vi "FRIC_navX_Internal_Serial_ProcessingLoop.vi"(7 "Device Number":T1, 9 "Stream Type":T2=enum."AHRSAndPositioning", 10 "Serial Port":T3=enum."MXP TTL", 11 "Update Rate (4Hz-200Hz)":u8=50 min=4 max=200) -> ()   [LabVIEW 2015]
doc: "This navX VI handles the reading/writing for the navX. All of the good stuff is in here.\nTHIS VI SHOULD NOT BE CALLED BY THE USER!"
uses:
  _NI WPI Serial USB/WPI_SerialPort_USB.ctl
  _TypeDefs/Z900_navX_SerialStreamTypeDef.ctl
  _TypeDefs/FRIC_navX_DeviceNumbersTypeDef.ctl
  _TypeDefs/FRIC_navX_I2C Process Loop TypeDef.ctl
  _TypeDefs/FRIC_navX_ProcessingLoopStatesTypeDef_I2C.ctl
  _TypeDefs/Z900_navX_DeviceTypeDef.ctl
  _TypeDefs/Z900_navX_ProtocolTypeDef.ctl
  _TypeDefs/Z900_navX_NotifyPacketTypeDef.ctl
  _TypeDefs/Z900_navX_ActionTypeDef.ctl
  <vilib>/Rock Robotics/SystemInterfaces/i2clib/i2c_bus.ctl
  _TypeDefs/Z900_navX_IntegrationControlRegisters.ctl
  <vilib>/Rock Robotics/WPI/SPI/WPI_SPIDevRef.ctl
  <vilib>/Rock Robotics/SystemInterfaces/spilib/spi_bus.ctl
  <vilib>/Rock Robotics/WPI/SerialPort/WPI_SerialPortRef.ctl
  _Device/_Internal/SERIAL/Z900_navX_SERIAL_ValidatePacketChecksum.vi
  _Device/_Internal/SERIAL/Z900_navX_SERIAL_ValidatePacketTermination.vi
  <vilib>/Rock Robotics/SystemInterfaces/Utilities/FPGA_UtilitiesRead LocalTime.vi
  _NI WPI Serial USB/_NI WPI Serial USB.lvlib
panel:
  out "Loop Time (ms)":dbl
  out "Connected":bool
  in  "Halt":bool
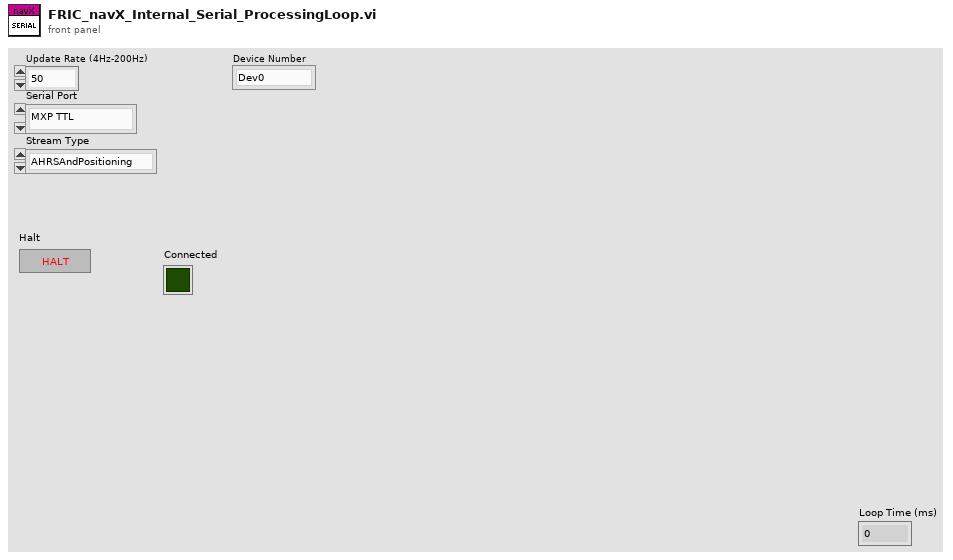
[diagram p1: front panel]
types:
  T1 = typedef "FRIC_navX_DeviceNumbersTypeDef.ctl" = enum16{"Dev0", "Dev1", "Dev2", "Dev3", "Dev4", "Dev5", "Dev6", "Dev7", "Dev8", "Dev9", "Dev10"}
  T2 = typedef "Z900_navX_SerialStreamTypeDef.ctl" = enum16{"YRPH", "Quaterinons", "Gyro/Raw", "AHRS", "AHRSAndPositioning"}
  T3 = typedef "_NI WPI Serial USB.lvlib/WPI_SerialPort_USB.ctl" = enum16{"Onboard RS-232", "MXP TTL", "USB"}
  T4 = typedef "FRIC_navX_I2C Process Loop TypeDef.ctl" = cluster{"State Array":T5[], "error":errorcluster, "FPGA Cluster":cluster{"Last Valid FPGA Time":dbl, "Error Count":i32, "Initialized":bool}, "Device Info":T6, "I2CDevRef":cluster{"DevStatus":errorcluster, "Device Address":u8, "Handle":i32, "I2C Bus":T8}, "Registry":u8[], "Command Array":T9[], "Connected?":bool, "navX Device Memory Size":i32, "notification":T10, "Memory Size Set":bool, "SPIDevRef":T12, "navX Serial Open":cluster{"Serial Port":T3, "Stream Type":T2}, "SerialPortRef":T14, "Serial Read Buffer":string, "Serial Write Buffer":string[], "Device Number":T1, "navX SPI Open":cluster{"SPI Bus":T13, "Clock Rate (Hz)":dbl}}
  T5 = typedef "FRIC_navX_ProcessingLoopStatesTypeDef_I2C.ctl" = enum16{"Process", "INI", "Check Packets Valid", "Close", "Flush Serial", "Generate Command", "Last Packet Valid", "Open", "Read", "Reset Serial", "Set Termination Char", "Update AE", "Wait", "Write", "Exit"}
  T6 = typedef "Z900_navX_DeviceTypeDef.ctl" = cluster{"Interface":cluster{"Protocol":T7, "Update Rate (4Hz-200Hz)":u8, "navX Open TypeDef":variant}, "Notify Packet":refnum<notifier>, "Loop VI Refnum":refnum<vi>, "Ready to Close Occurrence Refnum":refnum<k4>, "Name":string}
  T7 = typedef "Z900_navX_ProtocolTypeDef.ctl" = enum16{"SERIAL", "I2C", "SPI"}
  T8 = typedef "i2c_bus.ctl" = enum16{"I2C On-Board", "I2C MXP", "Invalid"}
  T9 = typedef "Z900_navX_IntegrationControlRegisters.ctl" = u8
  T10 = typedef "Z900_navX_NotifyPacketTypeDef.ctl" = cluster{"navX Action":T11, "Data":variant, "Stream Type":T2}
  T11 = typedef "Z900_navX_ActionTypeDef.ctl" = enum16{"None", "Halt", "Normal Read", "Update Serial Protocol", "Update Rate Htz", "Zero-Yaw", "Zero-Displacement", "Zero-Velocity"}
  T12 = typedef "WPI_SPIDevRef.ctl" = cluster{"DevStatus":errorcluster, "Handle":i32, "SPI Bus":T13}
  T13 = typedef "spi_bus.ctl" = enum16{"SPI On-Board, CS0", "SPI On-Board, CS1", "SPI On-Board, CS2", "SPI On-Board, CS3", "SPI MXP", "Invalid"}
  T14 = typedef "WPI_SerialPortRef.ctl" = cluster{"DevStatus":errorcluster, "Serial Port Name":refnum<visa-resource-name>}
  T15 = cluster{"Last Valid FPGA Time":dbl, "Error Count":i32, "Initialized":bool}
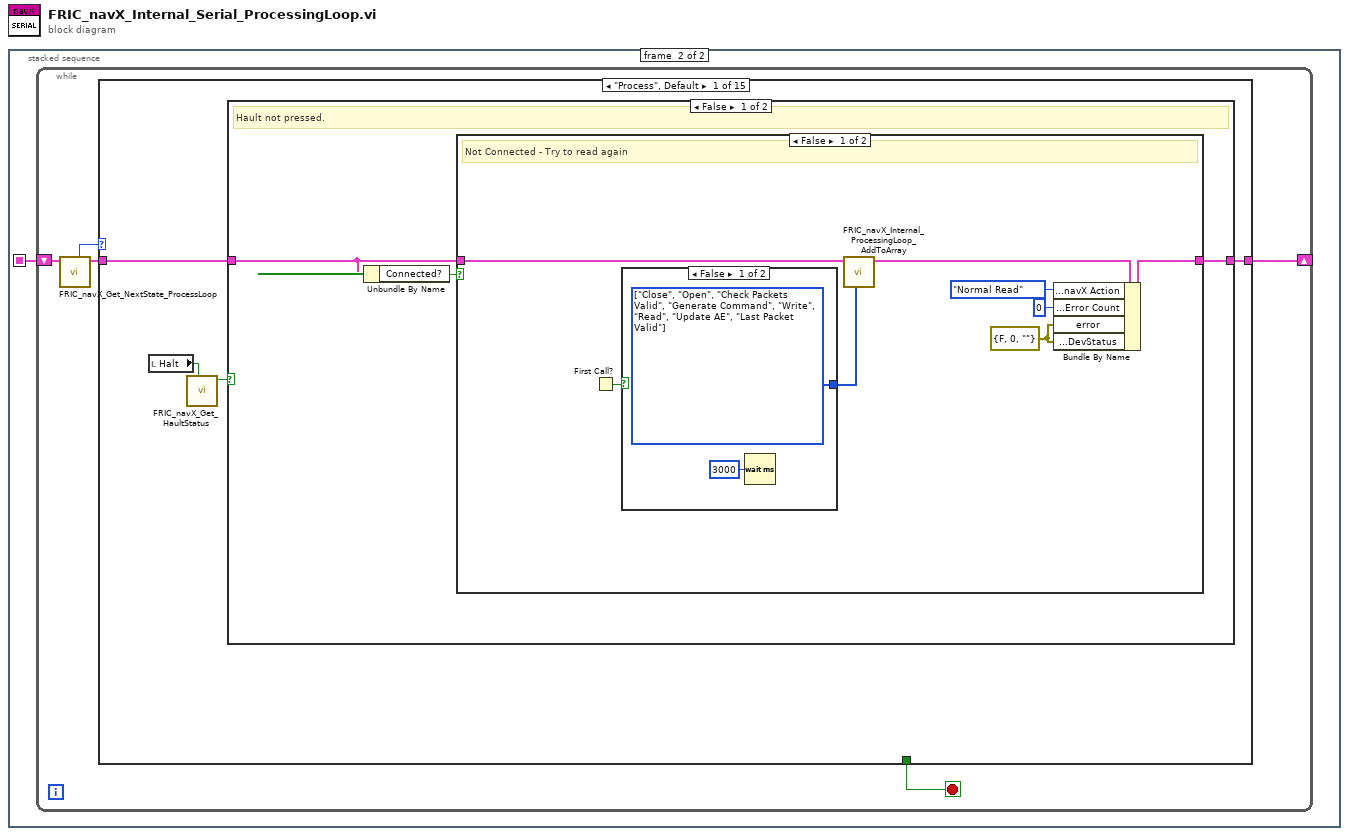
[diagram p0: block diagram]
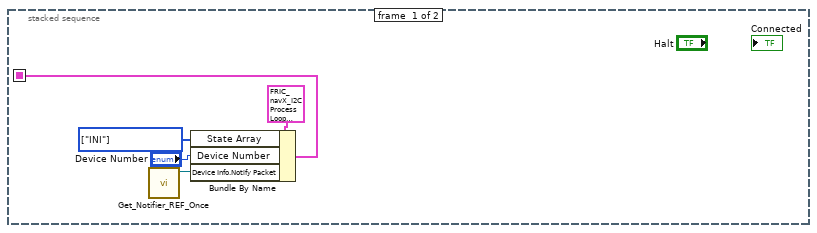
[diagram p2: hidden frame]
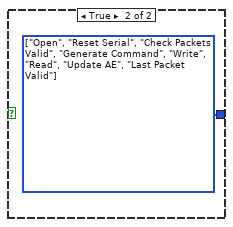
[diagram p3: hidden frame]
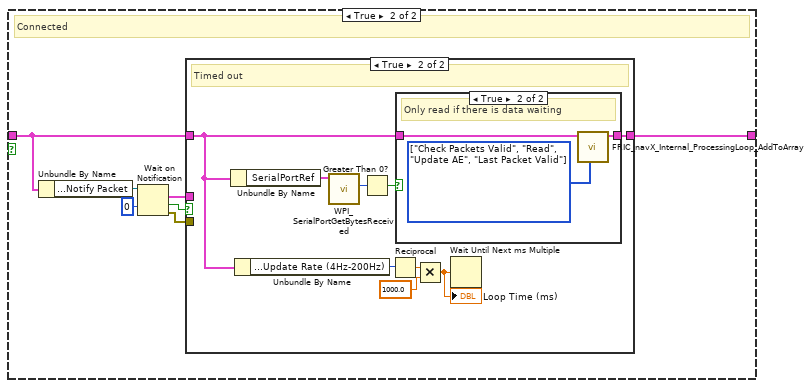
[diagram p4: hidden frame]
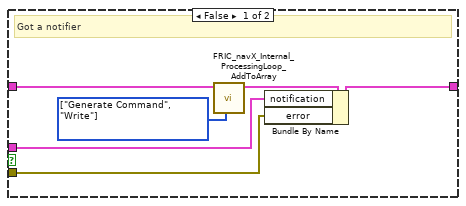
[diagram p5: hidden frame]
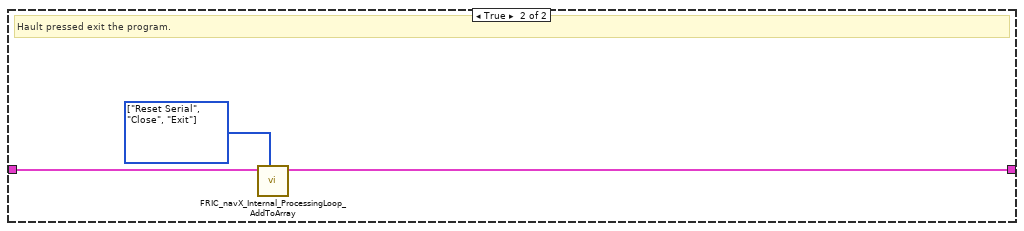
[diagram p7: hidden frame]
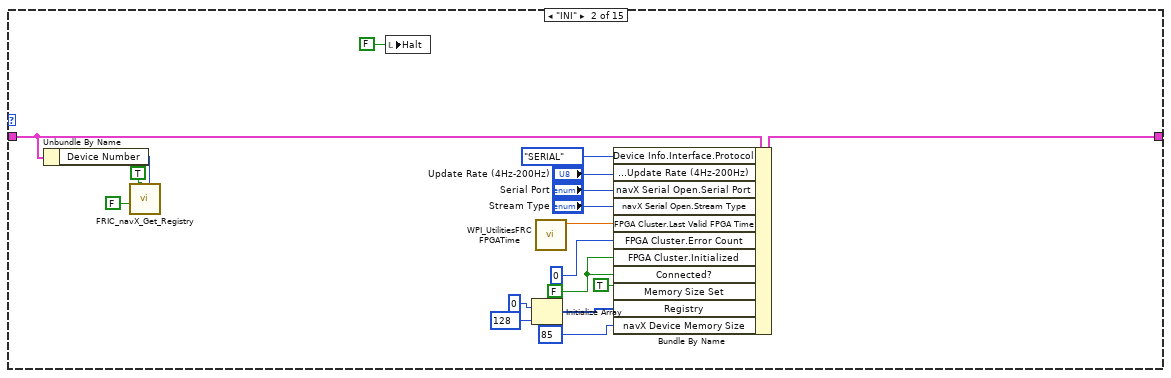
[diagram p8: hidden frame]
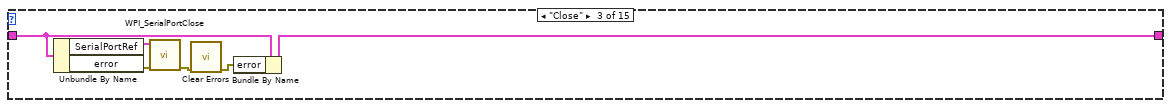
[diagram p9: hidden frame]
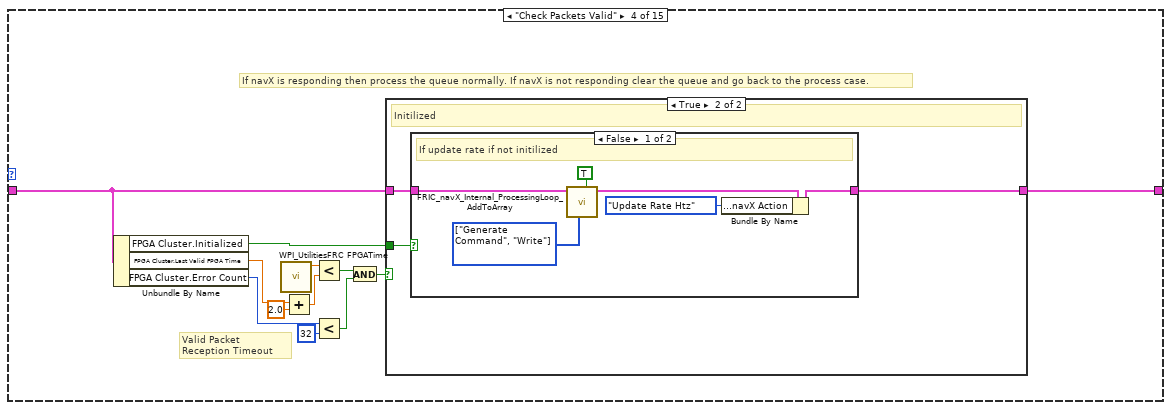
[diagram p10: hidden frame]
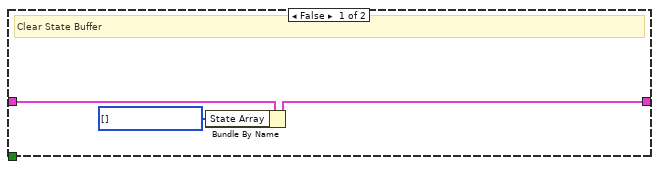
[diagram p11: hidden frame]
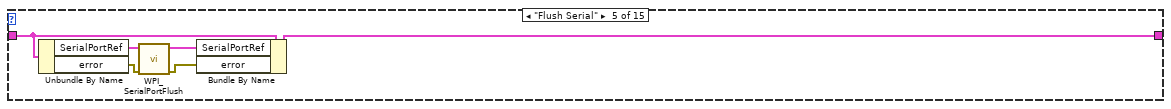
[diagram p13: hidden frame]
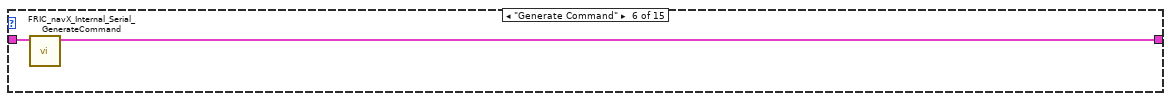
[diagram p14: hidden frame]
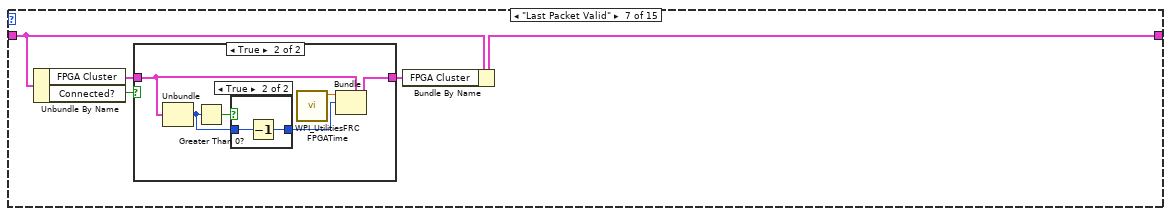
[diagram p15: hidden frame]
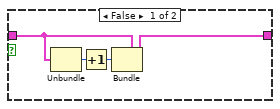
[diagram p16: hidden frame]
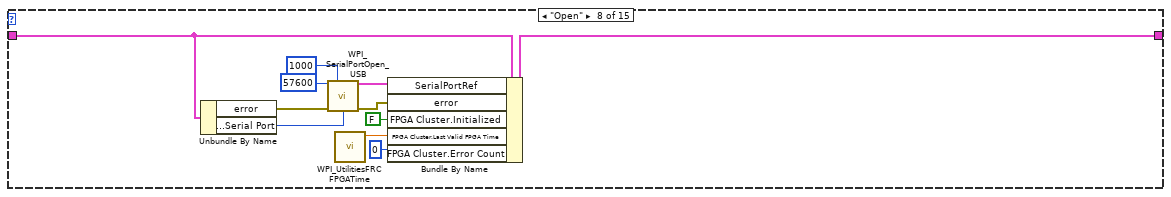
[diagram p18: hidden frame]
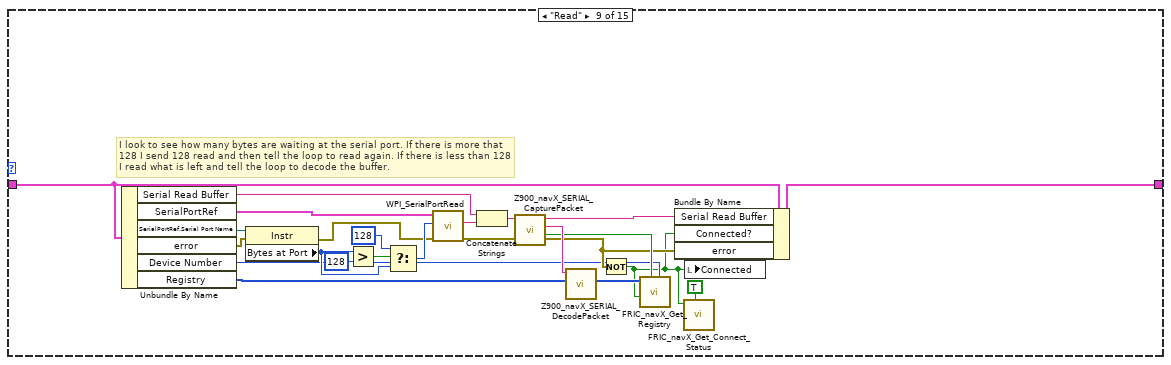
[diagram p19: hidden frame]
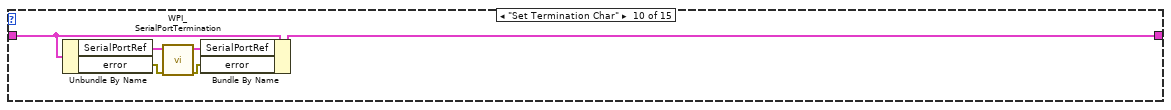
[diagram p20: hidden frame]
diagram:
  n1 = stacked-sequence {
    seq-local: [w5 _] -> [_ w6]
    frame #0 {
      w3 = T5[] [enum."INI"] items=["Process", "INI", "Check Packets Valid", "Close", "Flush Serial", "Generate Command", "Last Packet Valid", "Open", "Read", "Reset Serial", "Set Termination Char", "Update AE", "Wait", "Write", "Exit"] ("State Array")
      n2 = call "Get_Notifier_REF_Once.vi"() -> ("notifier ref out"=w1:refnum<notifier>)  [unwired: 10 in, 1 out]
      n3 = Bundle By Name(cluster=T4 {"State Array"=[enum."INI", enum."Open"], "error"={"status"=FALSE, "code"=0, "source"=""}, "FPGA Cluster"={"Last Valid FPGA Time"=0.0, "Error Count"=0, "Initialized"=FALSE}, "Device Info"={"Interface"={"Protocol"=enum."SERIAL", "Update Rate (4Hz-200Hz)"=4, "navX Open TypeDef"=variant}, "Notify Packet"=refnum, "Loop VI Refnum"=refnum, "Ready to Close Occurrence Refnum"=refnum, "Name"=""}, "I2CDevRef"={"DevStatus"={"status"=FALSE, "code"=0, "source"=""}, "Device Address"=0, "Handle"=0, "I2C Bus"=enum."Invalid"}, "Registry"=[], "Command Array"=[214, 32], "Connected?"=FALSE, "navX Device Memory Size"=85, "notification"={"navX Action"=enum."None", "Data"=variant, "Stream Type"=enum."YRPH"}, "Memory Size Set"=FALSE, "SPIDevRef"={"DevStatus"={"status"=FALSE, "code"=0, "source"=""}, "Handle"=0, "SPI Bus"=enum."SPI On-Board, CS0"}, "navX Serial Open"={"Serial Port"=enum."Onboard RS-232", "Stream Type"=enum."YRPH"}, "SerialPortRef"={"DevStatus"={"status"=FALSE, "code"=0, "source"=""}, "Serial Port Name"=""}, "Serial Read Buffer"="", "Serial Write Buffer"=[], "Device Number"=enum."Dev0", "navX SPI Open"={"SPI Bus"=enum."SPI MXP", "Clock Rate (Hz)"=500000.0}} ("I2C Process Loop TypeDef"), "State Array"=w3, "Device Number"="Device Number", "Device Info.Notify Packet"=w1) -> (w5:T4)
    }
    frame #1 {
      n4 = while {
        shift-right: [w7] -> _
        shift-left: w6 -> [w10]
        stop <- w11 stop-if-true
        n5 = call "FRIC_navX_Get_NextState_ProcessLoop.vi"("I2C Process Loop TypeDef (in)"=w10) -> ("I2C Process Loop TypeDef (out)"=w9:T4, "Current State"=w8:T5)  [unwired: 9 in]
        n6 = case shown="\"Process\", Default" w8 {
          tunnel: [_ _ _ _ _ _ _ _ _ _ _ _ _ TRUE _] -> w11
          tunnel: w9 -> [w14 w62 w82 w86 w109 w115 w119 w144 w150 w168 w178 w181 w196 w203 w210]
          tunnel: [w15 w69 w81 w87 w108 w114 w118 w143 w155 w169 w179 w181 w184 w203 w210] -> w7
          frame "Process", Default {
            n7 = local read "Halt"() -> (w13:bool)
            n8 = call "FRIC_navX_Get_HaultStatus.vi"("Update"=w13) -> ("Hault"=w12:bool)  [unwired: 10 in]
            n9 = case shown="False" w12 {
              tunnel: [w18 w57] -> w15
              tunnel: w14 -> [w16 w58]
              frame False {
                # "Hault not pressed."
                n10 = Unbundle By Name(w16) -> ("Connected?"=w17:bool)
                n11 = case shown="False" w17 {
                  tunnel: w16 -> [w26 w35]
                  tunnel: [w23 w36] -> w18
                  frame False {
                    w19 = errorcluster {"status"=FALSE, "code"=0, "source"=""} ("error")
                    # "Not Connected - Try to read again"
                    n12 = First Call?() -> (First Call?: T/F=w20:bool)
                    n13 = case shown="False" w20 {
                      tunnel: [w28 w29] -> w25
                      frame False {
                        w28 = T5[] [enum."Close", enum."Open", enum."Check Packets Valid", enum."Generate Command", enum."Write", enum."Read", enum."Update AE", enum."Last Packet Valid"] items=["Process", "INI", "Check Packets Valid", "Close", "Flush Serial", "Generate Command", "Last Packet Valid", "Open", "Read", "Reset Serial", "Set Termination Char", "Update AE", "Wait", "Write", "Exit"]
                        n14 = Wait (ms)(milliseconds to wait=u32 3000) -> ()  [unwired: 1 out]
                      }
                      frame True {
                        w29 = T5[] [enum."Open", enum."Reset Serial", enum."Check Packets Valid", enum."Generate Command", enum."Write", enum."Read", enum."Update AE", enum."Last Packet Valid"] items=["Process", "INI", "Check Packets Valid", "Close", "Flush Serial", "Generate Command", "Last Packet Valid", "Open", "Read", "Reset Serial", "Set Termination Char", "Update AE", "Wait", "Write", "Exit"]
                      }
                    }
                    n15 = call "FRIC_navX_Internal_ProcessingLoop_AddToArray.vi"("States Array"=w25, "I2C Process Loop TypeDef (in)"=w26) -> ("I2C Process Loop TypeDef (out)"=w24:T4)  [unwired: 9 in]
                    n16 = Bundle By Name(cluster=w24, "notification.navX Action"=Z900_navX_ActionTypeDef."Normal Read", "FPGA Cluster.Error Count"=0, "error"=w19, "SerialPortRef.DevStatus"=w19) -> (w23:T4)
                  }
                  frame True {
                    # "Connected"
                    n17 = Unbundle By Name(w35) -> ("Device Info.Notify Packet"=w34:refnum<notifier>)
                    n18 = Wait on Notification(notifier=w34, timeout in ms (-1)=0) -> (notification=w32:T10, timed out?=w30:bool, error out=w31:errorcluster)  [unwired: 2 in, 1 out]
                    n19 = case shown="True" w30 {
                      tunnel: w35 -> [w42 w43]
                      tunnel: [w41 w51] -> w36
                      tunnel: w32 -> [w40 _]
                      tunnel: w31 -> [w37 _]
                      frame False {
                        w38 = T5[] [enum."Generate Command", enum."Write"] items=["Process", "INI", "Check Packets Valid", "Close", "Flush Serial", "Generate Command", "Last Packet Valid", "Open", "Read", "Reset Serial", "Set Termination Char", "Update AE", "Wait", "Write", "Exit"] ("States Array")
                        # "Got a notifier"
                        n20 = call "FRIC_navX_Internal_ProcessingLoop_AddToArray.vi"("States Array"=w38, "I2C Process Loop TypeDef (in)"=w42) -> ("I2C Process Loop TypeDef (out)"=w39:T4)  [unwired: 9 in]
                        n21 = Bundle By Name(cluster=w39, "notification"=w40, "error"=w37) -> (w41:T4)
                      }
                      frame True {
                        # "Timed out"
                        n22 = Unbundle By Name(w43) -> ("SerialPortRef"=w50:T14)
                        n23 = Unbundle By Name(w43) -> ("Device Info.Interface.Update Rate (4Hz-200Hz)"=w44:u8)
                        n24 = call <vilib>:"WPI_SerialPortGetBytesReceived.vi"("SerialPortRef"=w50) -> ("Bytes at Port"=w49:u32)  [unwired: 8 in, 2 out]
                        n25 = Greater Than 0?(x=w49) -> (x > 0?=w48:bool)
                        n26 = Reciprocal(x=w44) -> (1/x=w45:dbl)
                        n27 = case shown="True" w48 {
                          tunnel: [w52 w54] -> w51
                          tunnel: w43 -> [w52 w53]
                          frame False {
                          }
                          frame True {
                            w55 = T5[] [enum."Check Packets Valid", enum."Read", enum."Update AE", enum."Last Packet Valid"] items=["Process", "INI", "Check Packets Valid", "Close", "Flush Serial", "Generate Command", "Last Packet Valid", "Open", "Read", "Reset Serial", "Set Termination Char", "Update AE", "Wait", "Write", "Exit"]
                            # "Only read if there is data waiting"
                            n28 = call "FRIC_navX_Internal_ProcessingLoop_AddToArray.vi"("States Array"=w55, "I2C Process Loop TypeDef (in)"=w53) -> ("I2C Process Loop TypeDef (out)"=w54:T4)  [unwired: 9 in]
                          }
                        }
                        n29 = Multiply(x=w45, y=1000.0) -> (x*y=w47:dbl)
                        "Loop Time (ms)" <- w47
                        n30 = Wait Until Next ms Multiple(millisecond multiple=w47) -> ()  [unwired: 1 out]
                      }
                    }
                  }
                }
              }
              frame True {
                w56 = T5[] [enum."Reset Serial", enum."Close", enum."Exit"] items=["Process", "INI", "Check Packets Valid", "Close", "Flush Serial", "Generate Command", "Last Packet Valid", "Open", "Read", "Reset Serial", "Set Termination Char", "Update AE", "Wait", "Write", "Exit"] ("States Array")
                # "Hault pressed exit the program."
                n31 = call "FRIC_navX_Internal_ProcessingLoop_AddToArray.vi"("States Array"=w56, "I2C Process Loop TypeDef (in)"=w58) -> ("I2C Process Loop TypeDef (out)"=w57:T4)  [unwired: 9 in]
              }
            }
          }
          frame "INI" {
            w67 = FALSE ("Initialized")
            n32 = Unbundle By Name(w62) -> ("Device Number"=w61:T1)
            n33 = call "FRIC_navX_Get_Registry.vi"("Device Number"=w61, "Update"=TRUE, "Connected?"=FALSE) -> ()  [unwired: 7 in, 2 out]
            n34 = local write "Halt"(FALSE ("Halt")) -> ()
            n35 = Initialize Array(u8 0 ("Received Data"), 128 ("hex")) -> (w65:u8[])
            n36 = call <vilib>:"WPI_UtilitiesFRC FPGATime.vi"() -> ("FPGA Time"=w71:dbl)  [unwired: 10 in, 1 out]
            n37 = Bundle By Name(cluster=w62, "Device Info.Interface.Protocol"=Z900_navX_ProtocolTypeDef."SERIAL" ("Protocol"), "Device Info.Interface.Update Rate (4Hz-200Hz)"="Update Rate (4Hz-200Hz)", "navX Serial Open.Serial Port"="Serial Port", "navX Serial Open.Stream Type"="Stream Type", "FPGA Cluster.Last Valid FPGA Time"=w71, "FPGA Cluster.Error Count"=0 ("Error Count"), "FPGA Cluster.Initialized"=w67, "Connected?"=w67, "Memory Size Set"=TRUE, "Registry"=w65, "navX Device Memory Size"=85 ("hex")) -> (w69:T4)
          }
          frame "Close" {
            n38 = Unbundle By Name(w82) -> ("SerialPortRef"=w79:T14, "error"=w78:errorcluster)
            n39 = call <vilib>:"WPI_SerialPortClose.vi"("error in (no error)"=w78, "SerialPortRef"=w79) -> ("error out"=w77:errorcluster)  [unwired: 9 in]
            n40 = call <vilib>:"Clear Errors.vi"("error in (no error)"=w77) -> ("error out"=w80:errorcluster)  [unwired: 5 in, 1 out]
            n41 = Bundle By Name(cluster=w82, "error"=w80) -> (w81:T4)
          }
          frame "Check Packets Valid" {
            # "If navX is responding then process the queue normally. If navX is not responding clear the queue and go back to the process case."
            # "Valid Packet Reception Timeout"
            n42 = Unbundle By Name(w86) -> ("FPGA Cluster.Initialized"=w84:bool, "FPGA Cluster.Last Valid FPGA Time"=w85:dbl, "FPGA Cluster.Error Count"=w83:i32)
            n43 = call <vilib>:"WPI_UtilitiesFRC FPGATime.vi"() -> ("FPGA Time"=w92:dbl)  [unwired: 10 in, 1 out]
            n44 = Add(x=w85, y=2.0) -> (x+y=w93:dbl)
            n45 = Less?(x=w92, y=w93) -> (x < y?=w90:bool)
            n46 = Less?(x=w83, y=32) -> (x < y?=w89:bool)
            n47 = And(x=w90, y=w89) -> (x .and. y?=w88:bool)
            n48 = case shown="True" w88 {
              tunnel: w86 -> [w97 w100]
              tunnel: [w96 w99] -> w87
              tunnel: w84 -> [_ w98]
              frame False {
                w95 = T5[] [] items=["Process", "INI", "Check Packets Valid", "Close", "Flush Serial", "Generate Command", "Last Packet Valid", "Open", "Read", "Reset Serial", "Set Termination Char", "Update AE", "Wait", "Write", "Exit"] ("f")
                # "Clear State Buffer"
                n49 = Bundle By Name(cluster=w97, "State Array"=w95) -> (w96:T4)
              }
              frame True {
                # "Initilized"
                n50 = case shown="False" w98 {
                  tunnel: w100 -> [w105 w107]
                  tunnel: [w103 w107] -> w99
                  frame False {
                    w101 = T5[] [enum."Generate Command", enum."Write"] items=["Process", "INI", "Check Packets Valid", "Close", "Flush Serial", "Generate Command", "Last Packet Valid", "Open", "Read", "Reset Serial", "Set Termination Char", "Update AE", "Wait", "Write", "Exit"] ("f")
                    # "If update rate if not initilized"
                    n51 = call "FRIC_navX_Internal_ProcessingLoop_AddToArray.vi"("Add to beginning"=TRUE, "States Array"=w101, "I2C Process Loop TypeDef (in)"=w105) -> ("I2C Process Loop TypeDef (out)"=w104:T4)  [unwired: 8 in]
                    n52 = Bundle By Name(cluster=w104, "notification.navX Action"=Z900_navX_ActionTypeDef."Update Rate Htz") -> (w103:T4)
                  }
                  frame True {
                    # "Everything is good keep going"
                  }
                }
              }
            }
          }
          frame "Flush Serial" {
            n53 = Unbundle By Name(w109) -> ("SerialPortRef"=w113:T14, "error"=w112:errorcluster)
            n54 = call <vilib>:"WPI_SerialPortFlush.vi"("error in (no error)"=w112, "SerialPortRef"=w113) -> ("error out"=w110:errorcluster, "SerialPortRef"=w111:T14)  [unwired: 8 in]
            n55 = Bundle By Name(cluster=w109, "SerialPortRef"=w111, "error"=w110) -> (w108:T4)
          }
          frame "Generate Command" {
            n56 = call "FRIC_navX_Internal_Serial_GenerateCommand.vi"("Serial Process Loop TypeDef (in)"=w115) -> ("Serial Process Loop TypeDef (out)"=w114:T4)  [unwired: 10 in]
          }
          frame "Last Packet Valid" {
            n57 = Unbundle By Name(w119) -> ("FPGA Cluster"=w120:T15, "Connected?"=w116:bool)
            n58 = case shown="True" w116 {
              tunnel: [w123 w130] -> w117
              tunnel: w120 -> [w122 w126]
              frame False {
                n59 = Unbundle(w122) -> ("Error Count"=w121:i32)  [unwired: 2 out]
                n60 = Increment(x=w121) -> (x+1=w124:i32)
                n61 = Bundle(cluster=w122, "Error Count"=w124) -> (w123:T15)  [unwired: 2 in]
              }
              frame True {
                n62 = Unbundle(w126) -> ("Error Count"=w125:i32)  [unwired: 2 out]
                n63 = Greater Than 0?(x=w125) -> (x > 0?=w128:bool)
                n64 = case shown="True" w128 {
                  tunnel: [w131 w133] -> w127
                  tunnel: w125 -> [w131 w132]
                  frame False {
                  }
                  frame True {
                    n65 = Decrement(x=w132) -> (x-1=w133:i32)
                  }
                }
                n66 = call <vilib>:"WPI_UtilitiesFRC FPGATime.vi"() -> ("FPGA Time"=w129:dbl)  [unwired: 10 in, 1 out]
                n67 = Bundle(cluster=w126, "Last Valid FPGA Time"=w129, "Error Count"=w127) -> (w130:T15)  [unwired: 1 in]
              }
            }
            n68 = Bundle By Name(cluster=w119, "FPGA Cluster"=w117) -> (w118:T4)
          }
          frame "Open" {
            n69 = Unbundle By Name(w144) -> ("error"=w135:errorcluster, "navX Serial Open.Serial Port"=w134:T3)
            n70 = call "WPI_SerialPortOpen_USB.vi"("Baud Rate"=u32 57600, "Timeout Value (ms)"=u32 1000, "error in (no error)"=w135, "Serial Port"=w134) -> ("SerialPortRef"=w138:T14, "error out"=w139:errorcluster)  [unwired: 10 in]
            n71 = call <vilib>:"WPI_UtilitiesFRC FPGATime.vi"() -> ("FPGA Time"=w137:dbl)  [unwired: 10 in, 1 out]
            n72 = Bundle By Name(cluster=w144, "SerialPortRef"=w138, "error"=w139, "FPGA Cluster.Initialized"=FALSE ("Initialized"), "FPGA Cluster.Last Valid FPGA Time"=w137, "FPGA Cluster.Error Count"=0) -> (w143:T4)
          }
          frame "Read" {
            # "I look to see how many bytes are waiting at the serial port. If there is more that 128 I send 128 read and then tell the loop to read again. If there is less than 128 I read what is left and tell the loop to decode the buffer."
            n73 = Unbundle By Name(w150) -> ("Serial Read Buffer"=w163:string, "SerialPortRef"=w164:T14, "SerialPortRef.Serial Port Name"=w167:refnum<visa-resource-name>, "error"=w166:errorcluster, "Device Number"=w147:T1, "Registry"=w152:u8[])
            n74 = property class="Instr"(reference=w167, error in=w166) -> (error out=w157:errorcluster, "Bytes at Port"=w160:u32)  [unwired: 1 in]
            n75 = Greater?(x=w160, y=u32 128) -> (0:w156:bool)
            n76 = Select(t=u32 128 ("y"), s=w156, f=w160) -> (s? t:f=w158:u32)
            n77 = call <vilib>:"WPI_SerialPortRead.vi"("error in (no error)"=w157, "Num Bytes to Read"=w158, "SerialPortRef"=w164) -> ("error out"=w148:errorcluster, "Buffer"=w165:string)  [unwired: 6 in, 1 out]
            n78 = Concatenate Strings(w163, w165) -> (w162:string)
            n79 = call "Z900_navX_SERIAL_CapturePacket.vi"("Buffer"=w162) -> ("Packet Located"=w149:bool, "Packet"=w151:string, "Buffer"=w154:string)  [unwired: 7 in, 1 out]
            n80 = call "Z900_navX_SERIAL_DecodePacket.vi"("Data (in)"=w152, "Packet (in)"=w151) -> ("Data"=w153:u8[])  [unwired: 7 in, 2 out]
            n81 = Not(x=w148) -> (.not. x?=w145:bool)
            n82 = call "FRIC_navX_Get_Registry.vi"("Device Number"=w147, "Update"=w149, "Connected?"=w145, "Registry (in)"=w153) -> ()  [unwired: 6 in, 2 out]
            n83 = Bundle By Name(cluster=w150, "Serial Read Buffer"=w154, "Connected?"=w145, "error"=w148) -> (w155:T4)
            n84 = call "FRIC_navX_Get_Connect_Status.vi"("Update"=TRUE, "Connected"=w145) -> ()  [unwired: 9 in, 1 out]
            n85 = local write "Connected"(w145) -> ()
          }
          frame "Set Termination Char" {
            n86 = Unbundle By Name(w168) -> ("SerialPortRef"=w173:T14, "error"=w172:errorcluster)
            n87 = call <vilib>:"WPI_SerialPortTermination.vi"("error in (no error)"=w172, "SerialPortRef"=w173) -> ("error out"=w170:errorcluster, "SerialPortRef"=w171:T14)  [unwired: 8 in]
            n88 = Bundle By Name(cluster=w168, "SerialPortRef"=w171, "error"=w170) -> (w169:T4)
          }
          frame "Reset Serial" {
            n89 = Unbundle By Name(w178) -> ("SerialPortRef"=w177:T14, "error"=w175:errorcluster)
            n90 = call <vilib>:"WPI_SerialPortReset.vi"("error in (no error)"=w175, "SerialPortRef"=w177) -> ("error out"=w174:errorcluster, "SerialPortRef"=w176:T14)  [unwired: 8 in]
            n91 = Bundle By Name(cluster=w178, "SerialPortRef"=w176, "error"=w174) -> (w179:T4)
          }
          frame "Wait" {
            n92 = Wait (ms)(milliseconds to wait=u32 1) -> ()  [unwired: 1 out]
          }
          frame "Write" {
            w183 = T5[] [enum."Flush Serial"] items=["Process", "INI", "Check Packets Valid", "Close", "Flush Serial", "Generate Command", "Last Packet Valid", "Open", "Read", "Reset Serial", "Set Termination Char", "Update AE", "Wait", "Write", "Exit"] ("States Array")
            # "This adds a flush after any write so we don't always have to tell the array to flush."
            n93 = Unbundle By Name(w196) -> ("SerialPortRef"=w194:T14, "Serial Write Buffer"=w191:string[], "SerialPortRef.DevStatus"=w195:errorcluster)
            n94 = Delete From Array(array=w191, index=0) -> (deleted portion=w190:string, array with subset deleted=w187:string[])  [unwired: 1 in]
            n95 = call <vilib>:"WPI_SerialPortWrite.vi"("error in (no error)"=w195, "Buffer"=w190, "SerialPortRef"=w194) -> ("error out"=w193:errorcluster, "SerialPortRef"=w192:T14)  [unwired: 6 in, 1 out]
            n96 = Empty Array?(array=w187) -> (empty?=w186:bool)
            n97 = Bundle By Name(cluster=w196, "SerialPortRef"=w192, "error"=w193, "Serial Write Buffer"=w187) -> (w188:T4)
            n98 = case shown="False" w186 {
              tunnel: [w200 w201] -> w185
              tunnel: w188 -> [w199 w201]
              frame False {
                w198 = T5[] [enum."Write"] items=["Process", "INI", "Check Packets Valid", "Close", "Flush Serial", "Generate Command", "Last Packet Valid", "Open", "Read", "Reset Serial", "Set Termination Char", "Update AE", "Wait", "Write", "Exit"] ("States Array")
                # "Write again because buffer is not empty."
                n99 = call "FRIC_navX_Internal_ProcessingLoop_AddToArray.vi"("Add to beginning"=TRUE, "States Array"=w198, "I2C Process Loop TypeDef (in)"=w199) -> ("I2C Process Loop TypeDef (out)"=w200:T4)  [unwired: 8 in]
              }
              frame True {
                # "Process the rest of the state array"
              }
            }
            n100 = call "FRIC_navX_Internal_ProcessingLoop_AddToArray.vi"("Add to beginning"=TRUE, "States Array"=w183, "I2C Process Loop TypeDef (in)"=w185) -> ("I2C Process Loop TypeDef (out)"=w184:T4)  [unwired: 8 in]
          }
          frame "Exit" {
            n101 = Unbundle By Name(w203) -> ("Device Info"=w202:T6)
            n102 = in-place {
              in-place-border: [TRUE] -> w205
              in-place-border: w202 -> [w206]
              # "Set Occurence of Close"
              n103 = Unbundle By Name(w206) -> ("Ready to Close Occurrence Refnum"=w208:refnum<k4>)
              n104 = local write "Halt"(FALSE ("Halt")) -> ()
              n105 = Set Occurrence(w208) -> ()
            }
            n106 = Stop(stop? (T)=w205) -> ()
          }
          frame "Update AE" {
            n107 = Unbundle By Name(w210) -> ("Device Number"=w211:T1)
            n108 = call "FRIC_navX_Internal_ProcessingLoop_UpdateAE.vi"("Device Number"=w211) -> ()  [unwired: 5 in, 10 out]
          }
        }
      }
    }
  }
